vi "nanocal -- nuclear schottky fit V3.vi"() -> ()   [LabVIEW 2020] (continued)
                  n444 = Look In Map(map=w852, key=nameformattingitem."units") -> (value=w853:string)  [unwired: 1 in, 1 out]
                  n445 = Format Value(format string=w850, value (0)=w856) -> (output string=w855:string)  [unwired: 1 in]
                  n446 = Concatenate Strings(w859, "_" ("event data"), w855, w853, "_" ("event data")) -> (w860:string)
                }
                frame True {
                }
              }
            }
            "state of all selectors string" <- w803
          }
          frame "action: reset colors" {
            w871 = map{T1, u32} {}  # Size: 0
            n447 = local read "parameter"() -> (w878:T1[])
            n448 = local read "colors"() -> (w880:u32[])
            n449 = for {
              shift-right: [w883] -> w879
              shift-left: w871 -> [w884]
              tunnel: w878 -> [w882] mode=indexing
              tunnel: w880 -> [w881] mode=indexing
              n450 = Insert Into Map(map in=w884, key=w882, value=w881) -> (map out=w883:map{T1, u32})  [unwired: 2 out]
            }
            n451 = local write "color Map"(w879) -> ()
            n452 = Look In Map(map=w879, key=3-lorentzian-parameters."ζ" ("Plost: sweep window")) -> (value=w877:u32)  [unwired: 1 in, 1 out]
            n453 = Look In Map(map=w879, key=3-lorentzian-parameters."τ1" ("Plost: sweep window")) -> (value=w876:u32)  [unwired: 1 in, 1 out]
            n454 = Look In Map(map=w879, key=3-lorentzian-parameters."τS" ("Plost: sweep window")) -> (value=w875:u32)  [unwired: 1 in, 1 out]
            n455 = Look In Map(map=w879, key=3-lorentzian-parameters."τN" ("Plost: sweep window")) -> (value=w874:u32)  [unwired: 1 in, 1 out]
            n456 = Look In Map(map=w879, key=3-lorentzian-parameters."τC" ("Plost: sweep window")) -> (value=w873:u32)  [unwired: 1 in, 1 out]
            n457 = Look In Map(map=w879, key=3-lorentzian-parameters."κ0" ("Plost: sweep window")) -> (value=w872:u32)  [unwired: 1 in, 1 out]
            n458 = property on="ζ" class="Slide (strict)"("Fill Color"=w877) -> ()  [unwired: 2 in, 2 out]
            n459 = property on="T1" class="Slide (strict)"("Fill Color"=w876) -> ()  [unwired: 2 in, 2 out]
            n460 = property on="τS" class="Slide (strict)"("Fill Color"=w875) -> ()  [unwired: 2 in, 2 out]
            n461 = property on="τN" class="Slide (strict)"("Fill Color"=w874) -> ()  [unwired: 2 in, 2 out]
            n462 = property on="τC" class="Slide (strict)"("Fill Color"=w873) -> ()  [unwired: 2 in, 2 out]
            n463 = property on="κ0" class="Slide (strict)"("Fill Color"=w872) -> ()  [unwired: 2 in, 2 out]
          }
          frame "action: copy from math" {
            (unwired) 3-lorentzian-heat-response_action."dζ" ("derivative")
            n464 = local read "mathematica thing"() -> (w890:map{i32, map{T1, dbl}})
            n465 = local read "file index"() -> (w889:i32)
            n466 = Generate User Event(user event=w885, event data cluster="action: new sweep" ("event data")) -> ()  [unwired: 2 in, 2 out]
            n467 = Look In Map(map=w890, key=w889) -> (key not found?=w887:bool, value=w888:map{T1, dbl})  [unwired: 1 in]
            n468 = case shown="False" w887 {
              tunnel: w888 -> [w896 _]
              frame False {
                n469 = Look In Map(map=w896, key=3-lorentzian-parameters."ζ" ("Plost: sweep window")) -> (value=w897:dbl)  [unwired: 1 in, 1 out]
                n470 = Look In Map(map=w896, key=3-lorentzian-parameters."τ1" ("Plost: sweep window")) -> (value=w895:dbl)  [unwired: 1 in, 1 out]
                n471 = Look In Map(map=w896, key=3-lorentzian-parameters."τS" ("Plost: sweep window")) -> (value=w894:dbl)  [unwired: 1 in, 1 out]
                n472 = Look In Map(map=w896, key=3-lorentzian-parameters."τN" ("Plost: sweep window")) -> (value=w893:dbl)  [unwired: 1 in, 1 out]
                n473 = Look In Map(map=w896, key=3-lorentzian-parameters."τC" ("Plost: sweep window")) -> (value=w892:dbl)  [unwired: 1 in, 1 out]
                n474 = Look In Map(map=w896, key=3-lorentzian-parameters."κ0" ("Plost: sweep window")) -> (value=w891:dbl)  [unwired: 1 in, 1 out]
                n475 = local write "ζ"(w897) -> ()
                n476 = local write "T1"(w895) -> ()
                n477 = local write "τS"(w894) -> ()
                n478 = local write "τN"(w893) -> ()
                n479 = local write "τC"(w892) -> ()
                n480 = local write "κ0"(w891) -> ()
              }
              frame True {
              }
            }
          }
          frame "action: copy to math" {
            (unwired) 0.0
            (unwired) 0.0
            w914 = 0.0
            w909 = T1[] [enum."ζ", enum."τ1", enum."τS", enum."τN", enum."τC", enum."κ0", enum."m1", enum."m2", enum."m3", enum."T (K)", enum."B (T)", enum."θ (deg)"] items=["ζ", "τ1", "τS", "τN", "τC", "κ0", "m1", "m2", "m3", "T (K)", "B (T)", "θ (deg)", "side (S|R)", "change (B|T)"]
            n481 = local read "ζ"() -> (w923:dbl)
            n482 = local read "T1"() -> (w922:dbl)
            n483 = local read "τS"() -> (w921:dbl)
            n484 = local read "τN"() -> (w920:dbl)
            n485 = local read "τC"() -> (w919:dbl)
            n486 = local read "κ0"() -> (w918:dbl)
            n487 = local read "T (K)"() -> (w913:dbl)
            n488 = local read "B (T)"() -> (w912:dbl)
            n489 = local read "θ (deg)"() -> (w911:dbl)
            n490 = Build Array(w923, w922, w921, w920, w919, w918, w914, w914, w914, w913, w912, w911) -> (w910:dbl[])
            n491 = Generate User Event(user event=w924, event data cluster="action: replot colors" ("event data")) -> ()  [unwired: 2 in, 2 out]
            n492 = for {
              tunnel: w910 -> [w926] mode=indexing
              tunnel: w909 -> [w927] mode=indexing
              tunnel: [w927] -> w908 mode=indexing
              shift-right: [w928] -> w906
              shift-left: map{T1, dbl} {} ("Map") -> [w929]
              n493 = Insert Into Map(map in=w929, key=w927, value=w926) -> (map out=w928:map{T1, dbl})  [unwired: 2 out]
            }
            n494 = local read "mathematica thing"() -> (w917:map{i32, map{T1, dbl}})
            n495 = local read "file index"() -> (w916:i32)
            n496 = call "3-lorentzian-heat-response -- V4.vi"("action"=3-lorentzian-heat-response_action."calc m1m2m3", "Map IN"=w906) -> ("Map OUT"=w905:map{T1, dbl})  [unwired: 7 in, 2 out]
            n497 = in-place {
              in-place-border: w908 -> [w934]
              in-place-border: w905 -> [w930]
              n498 = in-place-map #2(w917, w916) -> (w933:map{T1, dbl})  [unwired: 1 in, 1 out]
              n499 = for {
                tunnel: w934 -> [w936] mode=indexing
                shift-right: [w938] -> w932
                shift-left: w933 -> [w939]
                shift-right: [w937] -> _
                shift-left: w930 -> [w937]
                n500 = Look In Map(map=w937, key=w936) -> (value=w935:dbl)  [unwired: 1 in, 1 out]
                n501 = Insert Into Map(map in=w939, key=w936, value=w935) -> (map out=w938:map{T1, dbl})  [unwired: 2 out]
              }
              n502 = in-place-map #2(w932, LVMapReplaceAction."Modify Entry only if found" ("action")) -> (w915:map{i32, map{T1, dbl}})  [unwired: 2 out]
            }
            n503 = local write "mathematica thing"(w915) -> ()
          }
          frame "action: exit" {
          }
          frame "action: read from file" {
            n504 = Generate User Event(user event=w977, event data cluster="action: new sweep" ("event data")) -> ()  [unwired: 2 in, 2 out]
            n505 = Unbundle("off\nRe\nIm") -> ("Numeric"=w960:dbl, "Numeric"=w959:dbl)
            n506 = Re/Im To Complex(1:w959, 2:w960) -> (0:w946:cdb)
            n507 = call "file - read-write - list of lines-V2.vi"("read/write control"=file_--_read-write_control."read", "file path"="Read from file") -> ("header OUT"=w943:string, "list of lines OUT"=w945:string[], "filename out"=w976:string)  [unwired: 7 in]
            n508 = local read "cursor x selector"() -> (w956:map{T1, dbl})
            n509 = call "filename-manage.vi"("filename-action"=filename-action."get name", "file name IN"=w976) -> ("string OUT"=w942:string)  [unwired: 7 in, 2 out]
            n510 = case shown="\"as is\", Default" "tr" {
              tunnel: [w982 w999 w1048 w1075] -> w970
              tunnel: [w981 w998 w1047 w1074] -> w962
              tunnel: w946 -> [w980 w1004 w1043 w1064]
              tunnel: w945 -> [w983 w1012 w1042 w1063]
              tunnel: w943 -> [_ w1013 _ _]
              tunnel: w942 -> [_ w1002 _ _]
              tunnel: "Read from file" -> [_ w1001 _ _]
              frame "as is", Default {
                n511 = for {
                  tunnel: w983 -> [w994] mode=indexing
                  tunnel: [w989] -> w984 mode=indexing if=w985
                  tunnel: [w988] -> w982 mode=indexing if=w985
                  w990 = 0.0
                  n512 = Scan From String(format string="%f%f%f", input string=w994, initial scan location=u32 0, default 1=w990, default 2=w990, default 3=w990) -> (offset past scan=w986:u32, output 1=w988:dbl, output 2=w992:dbl, output 3=w991:dbl)  [unwired: 1 in, 2 out]
                  n513 = Greater Than 0?(x=w986) -> (x > 0?=w985:bool)
                  n514 = Re/Im To Complex(1:w991, 2:w992) -> (0:w989:cdb)
                }
                n515 = Subtract(x=w984, y=w980) -> (x-y=w981:cdb[])
              }
              frame "raw nanocal" {
                (unwired) nanocal_raw_file_manage_action_V1."read R side" ("action")
                n516 = call "filename-manage.vi"("filename-action"=filename-action."get side", "file name IN"=w1002) -> ("number OUT"=w996:dbl, "filename OUT"=w1000:string)  [unwired: 7 in, 1 out]
                n517 = case shown="8000, Default" w996 {
                  tunnel: [nanocal_raw_file_manage_action_V1."read S side" ("action") nanocal_raw_file_manage_action_V1."read R side" ("action")] -> w995
                  frame 8000, Default {
                  }
                  frame 4000 {
                  }
                }
                n518 = call "nanocal_raw_file_manage_V1.vi"("action"=w995, "list of lines IN"=w1012, "header IN"=w1013) -> ("z (K/W)  OUT"=w1005:cdb[], "f (Hz) OUT"=w1006:dbl[])  [unwired: 6 in, 1 out]
                n519 = Subtract(x=w1005, y=w1004) -> (x-y=w1007:cdb[])
                n520 = call "array -- freq-voltage transformations.vi"("freq voltage action"=array_--_freq-voltage_transformations_action."add -ω", "z In"=w1007, "ω IN"=w1006) -> ("z out"=w1010:cdb[], "ω out"=w1011:dbl[])  [unwired: 7 in]
                n521 = call "array -- freq-voltage transformations.vi"("freq voltage action"=array_--_freq-voltage_transformations_action."sort ω", "z In"=w1010, "ω IN"=w1011) -> ("z out"=w998:cdb[], "ω out"=w999:dbl[])  [unwired: 7 in]
                n522 = case shown="True" "generate labview files" {
                  tunnel: w1001 -> [_ w1023]
                  tunnel: w1000 -> [_ w1028]
                  tunnel: w999 -> [_ w1018]
                  tunnel: w998 -> [_ w1017]
                  frame False {
                  }
                  frame True {
                    n523 = call "filename-manage.vi"("filename-action"=filename-action."get basename", "file name IN"=w1028) -> ("string OUT"=w1026:string)  [unwired: 7 in, 2 out]
                    n524 = for {
                      tunnel: w1018 -> [w1037] mode=indexing
                      tunnel: w1017 -> [w1039] mode=indexing
                      tunnel: [w1029] -> w1016 mode=indexing
                      w1031 = "    "
                      w1038 = 12
                      n525 = Complex To Re/Im(x + iy=w1039) -> (x=w1036:dbl, y=w1035:dbl)
                      n526 = Number To Fractional String(number=w1036, precision (6)=w1038) -> (F-format string=w1033:string)  [unwired: 2 in]
                      n527 = Number To Fractional String(number=w1037, precision (6)=w1038) -> (F-format string=w1034:string)  [unwired: 2 in]
                      n528 = Number To Fractional String(number=w1035, precision (6)=w1038) -> (F-format string=w1032:string)  [unwired: 2 in]
                      n529 = Concatenate Strings("", w1034, w1031, w1033, w1031, w1032, w1031) -> (w1029:string)
                    }
                    n530 = Concatenate Strings(w1026, "_labview_.dat") -> (w1024:string)
                    n531 = Strip Path(path=w1023) -> (stripped path=w1022:path)  [unwired: 1 out]
                    n532 = Build Path(base path=w1022, name or relative path=w1024) -> (appended path=w1021:path)
                    n533 = call "file - read-write - list of lines-V2.vi"("read/write control"=file_--_read-write_control."write all", "header IN"="f(Hz)\tReR(K/W)\tImR(K/W)", "list of lines IN"=w1016, "file path"=w1021) -> ()  [unwired: 5 in, 3 out]
                  }
                }
              }
              frame "add - ω" {
                n534 = for {
                  tunnel: w1042 -> [w1060] mode=indexing
                  tunnel: [w1055] -> w1044 mode=indexing if=w1051
                  tunnel: [w1054] -> w1040 mode=indexing if=w1051
                  w1056 = 0.0
                  n535 = Scan From String(format string="%f%f%f", input string=w1060, initial scan location=u32 0, default 1=w1056, default 2=w1056, default 3=w1056) -> (offset past scan=w1052:u32, output 1=w1054:dbl, output 2=w1058:dbl, output 3=w1057:dbl)  [unwired: 1 in, 2 out]
                  n536 = Greater Than 0?(x=w1052) -> (x > 0?=w1051:bool)
                  n537 = Re/Im To Complex(1:w1057, 2:w1058) -> (0:w1055:cdb)
                }
                n538 = Subtract(x=w1044, y=w1043) -> (x-y=w1041:cdb[])
                n539 = call "array -- freq-voltage transformations.vi"("freq voltage action"=array_--_freq-voltage_transformations_action."add -ω", "z In"=w1041, "ω IN"=w1040) -> ("z out"=w1049:cdb[], "ω out"=w1050:dbl[])  [unwired: 7 in]
                n540 = call "array -- freq-voltage transformations.vi"("freq voltage action"=array_--_freq-voltage_transformations_action."sort ω", "z In"=w1049, "ω IN"=w1050) -> ("z out"=w1047:cdb[], "ω out"=w1048:dbl[])  [unwired: 7 in]
              }
              frame "full rydh" {
                n541 = for {
                  tunnel: w1063 -> [w1087] mode=indexing
                  tunnel: [w1082] -> w1065 mode=indexing if=w1078
                  tunnel: [w1081] -> w1061 mode=indexing if=w1078
                  w1083 = 0.0
                  n542 = Scan From String(format string="%f%f%f", input string=w1087, initial scan location=u32 0, default 1=w1083, default 2=w1083, default 3=w1083) -> (offset past scan=w1079:u32, output 1=w1081:dbl, output 2=w1085:dbl, output 3=w1084:dbl)  [unwired: 1 in, 2 out]
                  n543 = Greater Than 0?(x=w1079) -> (x > 0?=w1078:bool)
                  n544 = Re/Im To Complex(1:w1084, 2:w1085) -> (0:w1082:cdb)
                }
                n545 = Subtract(x=w1065, y=w1064) -> (x-y=w1062:cdb[])
                n546 = call "array -- freq-voltage transformations.vi"("freq voltage action"=array_--_freq-voltage_transformations_action."2 x ω", "z In"=w1062, "ω IN"=w1061) -> ("z out"=w1069:cdb[], "ω out"=w1071:dbl[])  [unwired: 7 in]
                n547 = call "array -- freq-voltage transformations.vi"("freq voltage action"=array_--_freq-voltage_transformations_action."R-phase(deg) to Re-Im", "z In"=w1069, "ω IN"=w1071) -> ("z out"=w1068:cdb[], "ω out"=w1070:dbl[])  [unwired: 7 in]
                n548 = call "array -- freq-voltage transformations.vi"("freq voltage action"=array_--_freq-voltage_transformations_action."add -ω", "z In"=w1068, "ω IN"=w1070) -> ("z out"=w1076:cdb[], "ω out"=w1077:dbl[])  [unwired: 7 in]
                n549 = call "array -- freq-voltage transformations.vi"("freq voltage action"=array_--_freq-voltage_transformations_action."sort ω", "z In"=w1076, "ω IN"=w1077) -> ("z out"=w1074:cdb[], "ω out"=w1075:dbl[])  [unwired: 7 in]
              }
            }
            n550 = call "filename-manage.vi"("filename-action"=filename-action."get T", "file name IN"=w942) -> ("number OUT"=w955:dbl, "filename OUT"=w973:string)  [unwired: 7 in, 1 out]
            "T (K)" <- w955
            n551 = Insert Into Map(map in=w956, key=3-lorentzian-parameters."T (K)" ("Plost: sweep window"), value=w955) -> (map out=w954:map{T1, dbl})  [unwired: 2 out]
            n552 = call "filename-manage.vi"("filename-action"=filename-action."get deg", "file name IN"=w973) -> ("number OUT"=w951:dbl, "filename OUT"=w963:string)  [unwired: 7 in, 1 out]
            "θ (deg)" <- w951
            n553 = Insert Into Map(map in=w954, key=3-lorentzian-parameters."θ (deg)" ("Plost: sweep window"), value=w951) -> (map out=w953:map{T1, dbl})  [unwired: 2 out]
            n554 = call "filename-manage.vi"("filename-action"=filename-action."get ind", "file name IN"=w963) -> ("number OUT"=→"file index":dbl, "filename OUT"=w958:string)  [unwired: 7 in, 1 out]
            n555 = call "filename-manage.vi"("filename-action"=filename-action."get B", "file name IN"=w958) -> ("number OUT"=w950:dbl)  [unwired: 7 in, 2 out]
            "B (T)" <- w950
            n556 = Insert Into Map(map in=w953, key=3-lorentzian-parameters."B (T)" ("Plost: sweep window"), value=w950) -> (map out=w952:map{T1, dbl})  [unwired: 2 out]
            n557 = local write "cursor x selector"(w952) -> ()
            n558 = call "filter - complex - four.vi"("omega (Hz) in"=w970, "z in"=w962, "span"="cspan") -> ("omega out"=w969:dbl[], "z out"=w968:cdb[], "dz/domega out"=w967:cdb[])  [unwired: 9 in, 5 out]
            n559 = call "nanocal -- publish -- freq scan V2.vi"("publisher action"=publisher_action."set", "dz/dω IN (V)"=w967, "z IN (V)"=w968, "ω IN (Hz)"=w969) -> ()  [unwired: 5 in, 3 out]
          }
          frame "action: save freq scan" {
            n560 = local read "Freq sweep name template"() -> (w1093:T11)
            n561 = call "MFLI -- publish -- freq scan.vi"("publisher action"=publisher_action."get") -> ("Voltage out (V)"=w1089:cdb[], "Freq out (Hz)"=w1090:dbl[])  [unwired: 9 in]
            n562 = call "filename-manage.vi"("filename pattern"=w1093, "filename-action"=filename-action."uniquenum", "folder IN"="Save folder", "file name IN"="freq sweep file name") -> ("filename OUT"=w1092:string)  [unwired: 5 in, 2 out]
            n563 = call "KM_appendline -- freq sweep.vi"("freq"=w1090, "Vout(V)"=w1089, "Save frequency scan"="Save folder", "read/write control"=KM_file_--_read-write_control."append one line", "name or relative path"=w1092) -> ()  [unwired: 15 in]
            n564 = local write "freq sweep file name"(w1092) -> ()
          }
          frame "void", Default {
          }
        }
      }
    }
  }
  n565 = call "replace cursor - plot ref - V2.vi"("Plot ref in"=w25, "new X"=w24, "new  Y"=w24, "cursor index"=2, "cursor action"=cursor_action."write") -> ()  [unwired: 11 in, 4 out]
  n566 = local write "newton pause"(w21) -> ()
  n567 = control-ref of="Plot:  colors"() -> (w22:refnum<vi>)
  n568 = while "interface" {
    tunnel: w39 -> [w1101]
    tunnel: w28 -> [w1100]
    tunnel: w25 -> [w1098]
    tunnel: w22 -> [w1097]
    tunnel: w21 -> [_]
    stop <- w1099 stop-if-true
    n569 = event shown="[21] \"generate empty string from filelist\": Value Change" {
      selector: w1101 -> [_ _ _ _ _ _ _ _ _ _ _ _ _ _ _ _ _ _ _ _ _ _ _ _ _ _ _ _]
      dyn-events: _ -> [_ _ _ _ _ _ _ _ _ _ _ _ _ _ _ _ _ _ _ _ _ _ _ _ _ _ _ _]
      timeout: _ -> [_ _ _ _ _ _ _ _ _ _ _ _ _ _ _ _ _ _ _ _ _ _ _ _ _ _ _ _]
      tunnel: w1100 -> [w1102 _ w1114 w1116 _ w1145 w1147 w1150 w1155 w1156 w1158 w1160 w1163 _ w1169 w1209 _ w1237 w1240 w1243 w1246 w1249 w1252 w1262 w1274 _ w1324 w1327]
      tunnel: [_ _ _ _ _ _ _ _ "load! :l" _ _ _ _ _ _ _ _ _ _ _ _ _ _ _ _ _ _ _] -> _
      tunnel: [_ _ _ _ _ _ _ _ _ _ _ _ _ _ _ _ _ _ _ _ _ _ _ _ _ w1278 _ _] -> w1099
      tunnel: [_ _ _ _ _ "go!" _ _ _ _ _ _ "parse! :p" _ _ _ "pause!" "uco! :u" "Read  τ's  from  Math !" "Write τ's to  Math!" "Math --> string OUT!" "generate empty string from filelist" "string IN  --> Math!" _ _ _ "plot landscape!" _] -> _
      tunnel: w1098 -> [_ _ _ _ _ _ _ _ _ _ _ _ _ _ w1165 _ _ _ _ _ _ _ _ _ _ _ _ _]
      tunnel: w1097 -> [_ _ _ _ _ _ _ _ _ _ _ _ _ _ _ w1232 _ _ _ _ _ _ _ _ _ _ _ _]
      event "Plot: sweep window": Cursor Move {
        n570 = event-data() -> ("CursIdx"=w1103:i32)  [unwired: 1 in]
        n571 = case shown="0..2" w1103 {
          tunnel: w1102 -> [w1105 _]
          frame 0..2 {
            w1104 = "action: fit"  # action
            n572 = Generate User Event(user event=w1105, event data cluster=w1104) -> ()  [unwired: 2 in, 2 out]
          }
          frame 3..5, Default {
          }
        }
      }
      event "scale gauge: Plot: complex plane": Value Change {
        n573 = event-data() -> ()  [unwired: 1 in, 1 out]
        n574 = local read "scale gauge: Plot: complex plane"() -> (w1112:dbl)
        n575 = control-ref of="Plot: sweep window"() -> (w1111:refnum<vi>)
        n576 = Multiply(x=w1112, y=0.3) -> (x*y=w1113:dbl)
        n577 = Bundle By Name(cluster=T27 {"window y"=0.0021014740628288917, "center x"=44850.89441339177, "center y"=2.5658109925320947, "window x"=17480.201988350764} ("window IN"), "window x"=w1112, "window y"=w1112, "center x"=w1113, "center y"=0.0) -> (w1110:T27)
        n578 = call "replace cursor - plot ref - V2.vi"("Plot ref in"=w1111, "window IN"=w1110, "cursor action"=cursor_action."zoom to win") -> ()  [unwired: 13 in, 4 out]
      }
      event "ζ", "T1", "τS", "τN", "τC", "κ0": Value Change {
        n579 = event-data() -> ()  [unwired: 1 in, 1 out]
        n580 = Generate User Event(user event=w1114, event data cluster="action: new sweep" ("event data")) -> ()  [unwired: 2 in, 2 out]
      }
      event Value Change {
        n581 = event-data() -> ()  [unwired: 1 in, 6 out]
        n582 = Generate User Event(user event=w1116, event data cluster="action: update enums" ("event data")) -> ()  [unwired: 2 in, 2 out]
      }
